vi "myRIO_BRig_RT_dataTrial_LC_ENL1_Trial.vi"() -> (2 "output_LC_ENL1_Trial":i32)   [LabVIEW 2014]
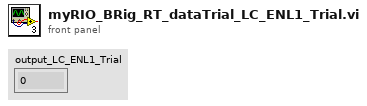
[diagram p1: front panel]
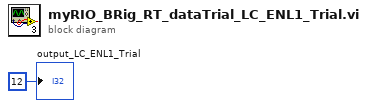
[diagram p0: block diagram]
diagram:
  "output_LC_ENL1_Trial" <- 12 ("output_iBlock")
